vi "Agilent PWM Get Stimulus.vi"(7 "Agilent PWM":T2, 8 "error in (no error)":errorcluster, 11 "VISA Resource Name":refnum<visa-resource-name>) -> (0 "error out":errorcluster, 2 "PWM Stimulus":T1, 3 "dup VISA Resource Name":refnum<visa-resource-name>)   [LabVIEW 2011]
uses:
  PWM Parameters.ctl
  TypeDefs/Agilent PWM Instrument Info.ctl
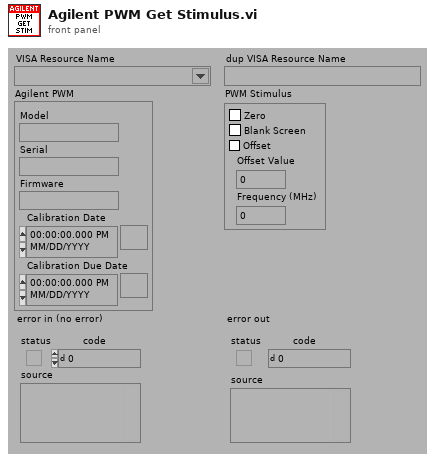
[diagram p1: front panel]
types:
  T1 = typedef "PWM Parameters.ctl" = cluster{"Zero":bool, "Blank Screen":bool, "Offset":bool, "Offset Value":dbl, "Frequency (MHz)":dbl}
  T2 = typedef "Agilent PWM Instrument Info.ctl" = cluster{"Model":string, "Serial":string, "Firmware":string, "Calibration Date":timestamp, "Calibration Due Date":timestamp}
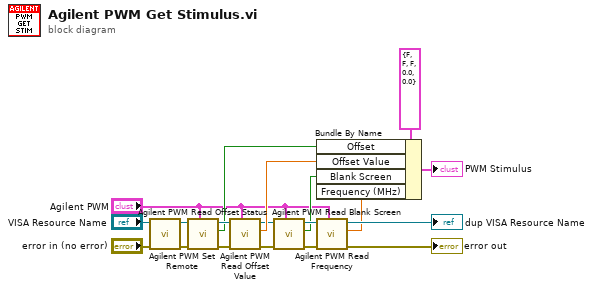
[diagram p0: block diagram]
diagram:
  n1 = call "Agilent PWM Set Remote.vi"("error in (no error)"="error in (no error)", "VISA Resource Name"="VISA Resource Name") -> ("error out"=w12:errorcluster, "dup VISA Resource Name"=w13:refnum<visa-resource-name>)  [unwired: 8 out]
  n2 = call "Agilent PWM Read Offset Status.vi"("Agilent PWM"="Agilent PWM", "error in (no error)"=w12, "VISA Resource Name"=w13) -> ("error out"=w17:errorcluster, "On/Off"=w11:bool, "dup VISA Resource Name"=w16:refnum<visa-resource-name>)  [unwired: 6 out]
  n3 = call "Agilent PWM Read Offset Value.vi"("Agilent PWM"="Agilent PWM", "error in (no error)"=w17, "VISA Resource Name"=w16) -> ("error out"=w8:errorcluster, "Value (dB)"=w10:dbl, "dup VISA Resource Name"=w9:refnum<visa-resource-name>)  [unwired: 1 in, 5 out]
  n4 = call "Agilent PWM Read Blank Screen.vi"("Agilent PWM"="Agilent PWM", "error in (no error)"=w8, "VISA Resource Name"=w9) -> ("error out"=w7:errorcluster, "Blank Screen"=w2:bool, "dup VISA Resource Name"=w6:refnum<visa-resource-name>)  [unwired: 6 out]
  n5 = call "Agilent PWM Read Frequency.vi"("Agilent PWM"="Agilent PWM", "error in (no error)"=w7, "VISA Resource Name"=w6) -> ("error out"=→"error out":errorcluster, "Frequency (MHz)"=w3:dbl, "dup VISA Resource Name"=→"dup VISA Resource Name":refnum<visa-resource-name>)  [unwired: 6 in]
  n6 = Bundle By Name(cluster=T1 {"Zero"=FALSE, "Blank Screen"=FALSE, "Offset"=FALSE, "Offset Value"=0.0, "Frequency (MHz)"=0.0} ("Stimulus"), "Offset"=w11, "Offset Value"=w10, "Blank Screen"=w2, "Frequency (MHz)"=w3) -> (→"PWM Stimulus":T1)
